vi "Configure Waveform (Ramp).vi"(0 "VISA resource name":refnum<visa-resource-name>, 1 "Frequency (1000 Hz)":dbl=1000.0, 5 "Ramp Symmetry (100 %)":i32=100 min=0 max=100, 9 "Amplitude (1.0 Vpp)":dbl=1.0, 11 "error in (no error)":errorcluster, 12 "DC Offset (0.00 V)":dbl) -> (4 "VISA resource name out":refnum<visa-resource-name>, 15 "error out":errorcluster)   [LabVIEW 2017, in "Keithley 3390.lvlib"]
doc: "Sets the waveform parameters for a ramp waveform and makes it the active waveform function."
uses:
  Keithley 3390.lvlib
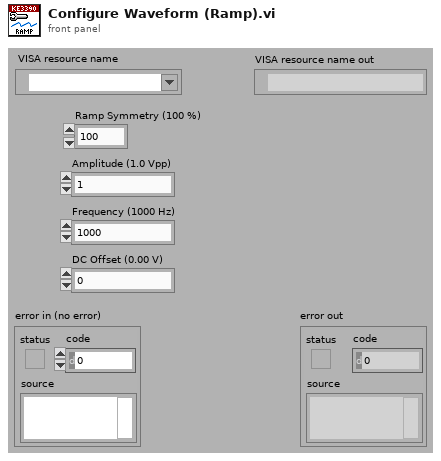
[diagram p1: front panel]
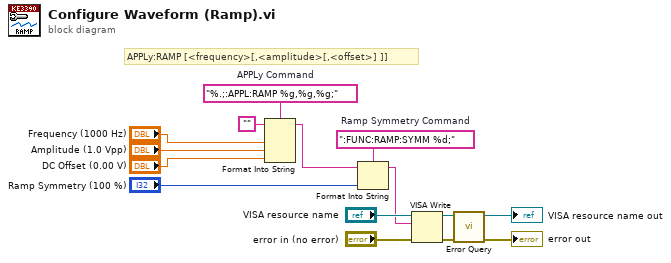
[diagram p0: block diagram]
diagram:
  w7 = "%.;:APPL:RAMP %g,%g,%g;"  # APPLy Command
  w9 = ":FUNC:RAMP:SYMM %d;"  # Ramp Symmetry Command
  # "APPLy:RAMP [<frequency>[,<amplitude>[,<offset>] ]]"
  n1 = Format Into String(format string=w7, initial string="", "Frequency (1000 Hz)", "Amplitude (1.0 Vpp)", "DC Offset (0.00 V)") -> (resulting string=w5:string)  [unwired: 1 in, 1 out]
  n2 = Format Into String(format string=w9, initial string=w5, "Ramp Symmetry (100 %)") -> (resulting string=w6:string)  [unwired: 1 in, 1 out]
  n3 = VISA Write(VISA resource name="VISA resource name", write buffer=w6, error in (no error)="error in (no error)") -> (VISA resource name out=w11:refnum<visa-resource-name>, error out=w10:errorcluster)  [unwired: 1 out]
  n4 = call "Error Query.vi"("error in (no error)"=w10, "VISA resource name"=w11) -> ("error out"=→"error out":errorcluster, "VISA resource name out"=→"VISA resource name out":refnum<visa-resource-name>)  [unwired: 6 in, 2 out]
